vi "FPGA_AIReadAccumulatorDeadband.vi"(8 "error in (no error)":errorcluster, 10 "Channel":T1, 11 "AI Reference in":T2) -> (0 "error out":errorcluster, 1 "Deadband":i32, 3 "AI Reference out":T2)   [LabVIEW 2017]
uses:
  <vilib>/Rock Robotics/SystemInterfaces/AI/FPGA_AIDevRef.ctl
  <vilib>/Rock Robotics/SystemInterfaces/AI/FPGA_AIChannel.ctl
  <vilib>/Rock Robotics/SystemInterfaces/System/FPGA_SystemFPGA Ref Global.vi
  <vilib>/Utility/error.llb/Error Cluster From Error Code.vi
  <vilib>/rvi/errors/niLvFpgaAdjustHostInterfaceError.vi
  <vilib>/rvi/interface/nirviReadWriteControl/nirviReadWriteControl.xnode
  <vilib>/Rock Robotics/SystemInterfaces/System/FPGA_SystemFRC FPGA Ref.ctl
  NiFpgaLv.dll
  <vilib>/rvi/interface/Simulation/niFpgaSimulationCallBeginRW.vi
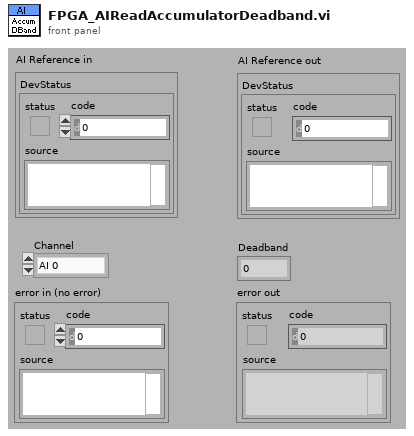
[diagram p1: front panel]
types:
  T1 = typedef "FPGA_AIChannel.ctl" = enum8{"AI 0", "AI 1", "AI 2", "AI 3", "AI MXP 0", "AI MXP 1", "AI MXP 2", "AI MXP 3", "Invalid"}
  T2 = typedef "FPGA_AIDevRef.ctl" = cluster{"DevStatus":errorcluster}
  T3 = typedef "FPGA_SystemFRC FPGA Ref.ctl" = refnum<k20>
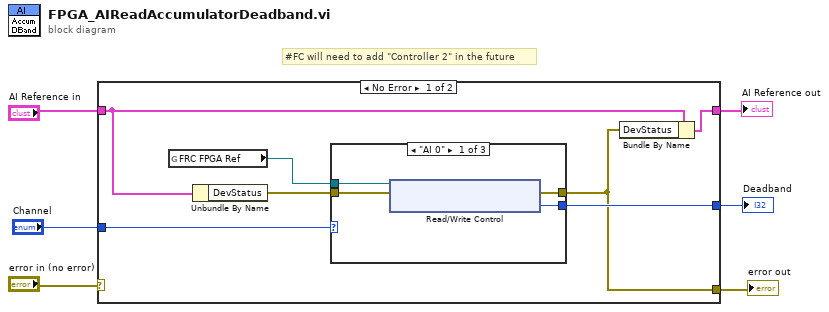
[diagram p0: block diagram]
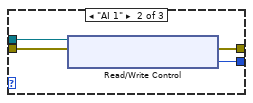
[diagram p2: hidden frame]
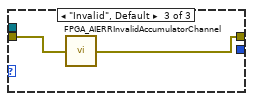
[diagram p3: hidden frame]
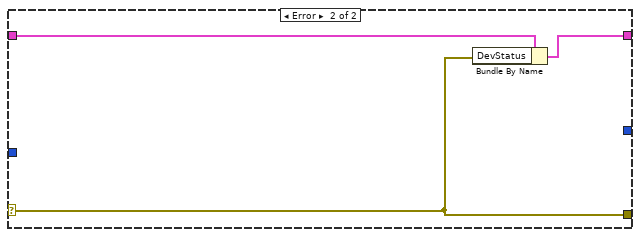
[diagram p4: hidden frame]
diagram:
  # "#FC will need to add \"Controller 2\" in the future"
  n1 = case shown="No Error" "error in (no error)" {
    selector: "error in (no error)" -> [_ w24]
    tunnel: [w13 w26] -> w5
    tunnel: "AI Reference in" -> [w12 w25]
    tunnel: [w9 w24] -> w3
    tunnel: [w10 _] -> w2
    tunnel: "Channel" -> [w8 _]
    frame No Error {
      n2 = global read "FPGA_SystemFPGA Ref Global.vi" "FRC FPGA Ref"() -> (w7:T3)
      n3 = Unbundle By Name(w12) -> ("DevStatus"=w11:errorcluster)
      n4 = case shown="\"AI 0\"" w8 {
        tunnel: w11 -> [w14 w19 w23]
        tunnel: [w17 w21 w22] -> w9
        tunnel: [w16 w20 _] -> w10
        tunnel: w7 -> [w15 w18 _]
        frame "AI 0" {
          n5 = xnode "Read/Write Control"("FPGA VI Reference In"=w15, "error in"=w14) -> ("error out"=w17:errorcluster, "Accumulator0.Deadband"=w16:i32)  [unwired: 1 out]
        }
        frame "AI 1" {
          n6 = xnode "Read/Write Control"("FPGA VI Reference In"=w18, "error in"=w19) -> ("error out"=w21:errorcluster, "Accumulator1.Deadband"=w20:i32)  [unwired: 1 out]
        }
        frame "Invalid", Default {
          n7 = call <vilib>:"FPGA_AIERRInvalidAccumulatorChannel.vi"("error in (no error)"=w23) -> ("error out"=w22:errorcluster)
        }
      }
      n8 = Bundle By Name(cluster=w12, "DevStatus"=w9) -> (w13:T2)
    }
    frame Error {
      n9 = Bundle By Name(cluster=w25, "DevStatus"=w24) -> (w26:T2)
    }
  }
  "AI Reference out" <- w5
  "error out" <- w3
  "Deadband" <- w2
